vi "Write rioResourceName.vi"(8 "error in (no error)":errorcluster, 10 "rioResourceName":string="RIO0", 11 "RIOConfig in":refnum<class "RIOConfig.lvclass">) -> (0 "error out":errorcluster, 3 "RIOConfig out":refnum<class "RIOConfig.lvclass">)   [LabVIEW 2013, in "ComponentData.lvlib" / "RIOConfig.lvclass"]
uses:
  <userlib>/Common/Component/common_application/RT/ComponentData/ConfigurationHandler/RIOConfig/RIOConfig.lvclass
  <userlib>/Common/Component/common_application/RT/ComponentData/ConfigurationHandler/RIOConfig/RIOConfig.lvclass/RIOConfig.ctl
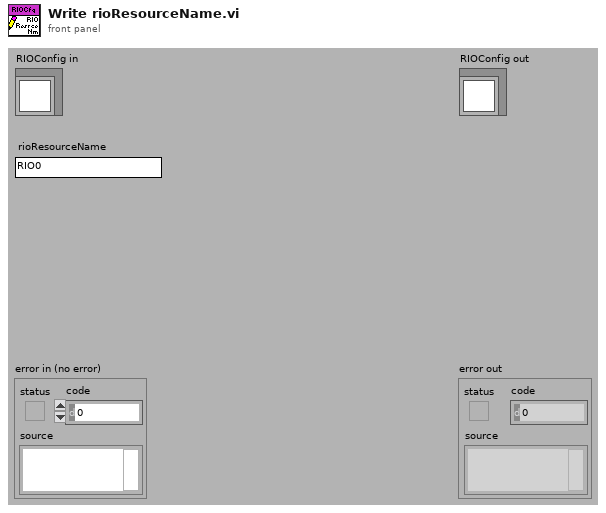
[diagram p1: front panel]
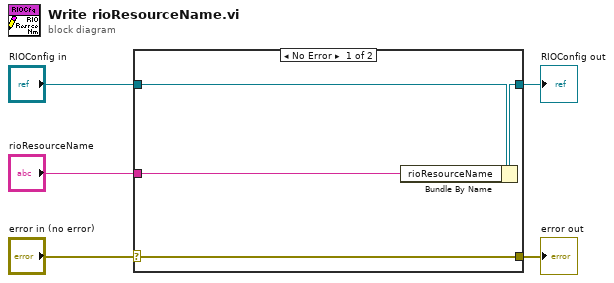
[diagram p0: block diagram]
diagram:
  n1 = case shown="No Error" "error in (no error)" {
    selector: "error in (no error)" -> [w9 w10]
    tunnel: [w9 w10] -> w4
    tunnel: [w7 w11] -> w2
    tunnel: "RIOConfig in" -> [w8 w11]
    tunnel: "rioResourceName" -> [w6 _]
    frame No Error {
      n2 = Bundle By Name(cluster=w8, "rioResourceName"=w6) -> (w7:refnum<class "RIOConfig.lvclass">)
    }
    frame Error {
    }
  }
  "error out" <- w4
  "RIOConfig out" <- w2
